vi "Lossy Enqueue.vi"(8 "error in (no error)":errorcluster, 10 "Data to Enqueue":refnum<class "Data.lvclass">, 11 "Queue in":refnum<class "Queue.lvclass">) -> (0 "error out":errorcluster, 1 "Overflow?":bool, 2 "Overflow element":refnum<class "Data.lvclass">, 3 "Queue out":refnum<class "Queue.lvclass">)   [LabVIEW 2020, in "Data.lvlib" / "Queue.lvclass"]
doc: "Enqueue a Data element on the queue front end of the queue."
uses:
  Queue.lvclass
  Data.lvclass
  Queue.lvclass/Queue.ctl
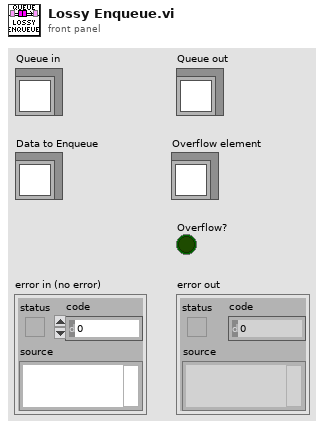
[diagram p1: front panel]
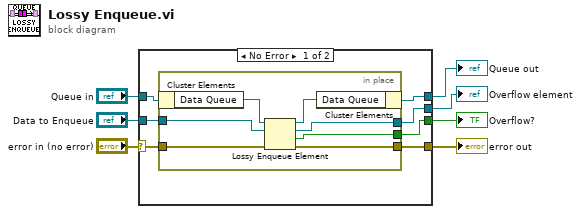
[diagram p0: block diagram]
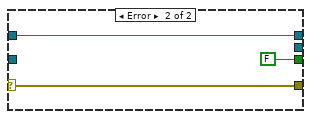
[diagram p2: hidden frame]
diagram:
  n1 = case shown="No Error" "error in (no error)" {
    selector: "error in (no error)" -> [w11 w24]
    tunnel: [w10 w24] -> w6
    tunnel: [w13 w23] -> w4
    tunnel: "Queue in" -> [w14 w23]
    tunnel: "Data to Enqueue" -> [w12 _]
    tunnel: [w9 FALSE ("timed out?")] -> w2
    tunnel: [w8 _] -> w1
    frame No Error {
      n2 = in-place {
        in-place-border: w12 -> [w19]
        in-place-border: w11 -> [w16]
        in-place-border: [w18] -> w10
        in-place-border: [w17] -> w9
        in-place-border: [w15] -> w8
        n3 = in-place-cluster #1(w14) -> ("Data Queue"=w21:refnum<queue>)
        n4 = Lossy Enqueue Element(queue=w21, element=w19, error in (no error)=w16) -> (queue out=w20:refnum<queue>, overflow element=w15:refnum<class "Data.lvclass">, overflow?=w17:bool, error out=w18:errorcluster)
        n5 = in-place-cluster #1("Data Queue"=w20) -> (w13:refnum<class "Queue.lvclass">)
      }
    }
    frame Error {
    }
  }
  "error out" <- w6
  "Queue out" <- w4
  "Overflow?" <- w2
  "Overflow element" <- w1
